vi "IsBitSetPresenceVector.vi"() -> ()   [LabVIEW 2009]
panel:
  out "result":bool
  in  "bit":i32
  in  "Presence Vector":u16 format="%b"
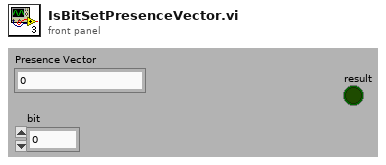
[diagram p1: front panel]
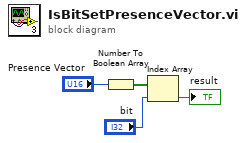
[diagram p0: block diagram]
diagram:
  n1 = Number To Boolean Array(number="Presence Vector") -> (Boolean array=w1:bool[])
  n2 = Index Array(array=w1, index="bit") -> (element=→"result":bool)
